vi "Write Teller Metadata.vi"(10 "Teller Metadata":refnum<class "Teller Metadata.lvclass">, 11 "Base Teller in":refnum<class "Base Teller.lvclass">) -> (3 "Base Teller out":refnum<class "Base Teller.lvclass">)   [LabVIEW 2020, in "jettl.lvlib" / "Base Teller.lvlib" / "Base Teller.lvclass"]
uses:
  Base Teller.lvclass
  Teller Metadata/Teller Metadata.lvclass
  Base Teller.lvclass/Base Teller.ctl
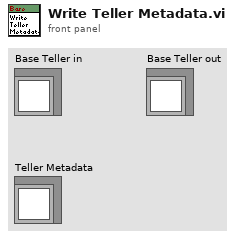
[diagram p1: front panel]
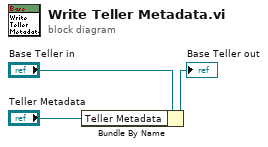
[diagram p0: block diagram]
diagram:
  n1 = Bundle By Name(cluster="Base Teller in", "Teller Metadata"="Teller Metadata") -> (→"Base Teller out":refnum<class "Base Teller.lvclass">)
